vi "SLSC Get Channel Properties.vi"(0 "Node Ptr":T1 format="%.0x", 11 "error in (no error)":errorcluster) -> (2 "Loop time (ms)":u32, 3 "Description":string, 4 "Section Ref out":T1 format="%.0x", 6 "Module Number":i32, 8 "Name":string, 10 "Device Version":string, 13 "Default Value":bool, 14 "Reset Value":bool, 15 "error out":errorcluster)   [LabVIEW 2020, in "SLSC EDS System Explorer.lvlib"]
uses:
  System Explorer/SLSC EDS System Explorer.lvlib
  <vilib>/NI VeriStand/Custom Device API/Custom Device Item Ref.ctl
  Shared/Constants.vi
  <vilib>/NI VeriStand/Custom Device API/Get Item Property (I32).vi
  <vilib>/NI VeriStand/Custom Device API/Get Item Property (Boolean).vi
  <vilib>/NI VeriStand/Custom Device API/Custom Device API.lvlib
  Shared/SLSC EDS Shared.lvlib
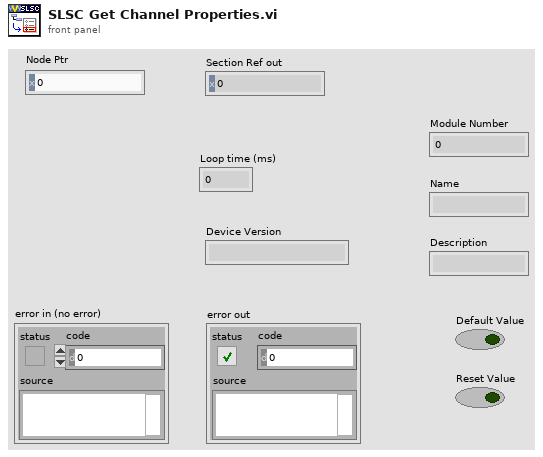
[diagram p1: front panel]
types:
  T1 = typedef "Custom Device API.lvlib/Custom Device Item Ref.ctl" = u64
  T2 = typedef "Custom Device API.lvlib/Custom Device Item Info.ctl" = cluster{"Name":string, "Is Channel":bool, "GUID":string, "Is Waveform":bool}
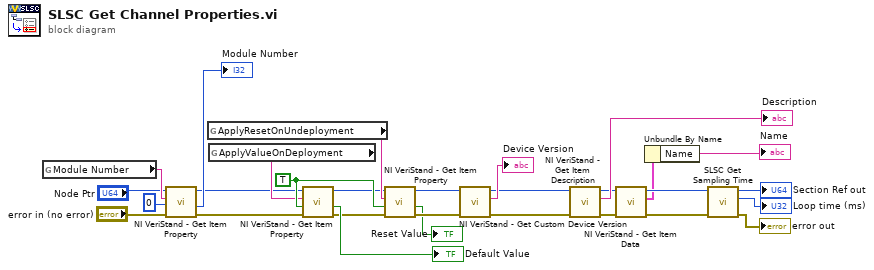
[diagram p0: block diagram]
diagram:
  w22 = TRUE ("Default Value")
  n1 = global read "Constants.vi" "Module Number"() -> (w13:string)
  n2 = call-poly <vilib>:"NI VeriStand - Get Item Property.vi"("error in (no error)"="error in (no error)", "Default Value"=0, "Property Name"=w13, "Item Ref in"="Node Ptr") -> ("error out"=w25:errorcluster, "Value"=→"Module Number":i32, "Item Ref out"=w15:T1)  [unwired: 4 in, 1 out]
  n3 = global read "Constants.vi" "ApplyResetOnUndeployment"() -> (w18:string)
  n4 = global read "Constants.vi" "ApplyValueOnDeployment"() -> (w16:string)
  n5 = call-poly <vilib>:"NI VeriStand - Get Item Property.vi"("error in (no error)"=w25, "Default Value"=w22, "Property Name"=w16, "Item Ref in"=w15) -> ("error out"=w19:errorcluster, "Value"=→"Default Value":bool, "Item Ref out"=w17:T1)  [unwired: 4 in, 1 out]
  n6 = call-poly <vilib>:"NI VeriStand - Get Item Property.vi"("error in (no error)"=w19, "Default Value"=w22, "Property Name"=w18, "Item Ref in"=w17) -> ("error out"=w29:errorcluster, "Value"=→"Reset Value":bool, "Item Ref out"=w28:T1)  [unwired: 4 in, 1 out]
  n7 = call <vilib>:"NI VeriStand - Get Custom Device Version.vi"("error in (no error)"=w29, "Device Ref in"=w28) -> ("error out"=w27:errorcluster, "Value"=→"Device Version":string, "Device Ref out"=w11:T1)  [unwired: 7 in]
  n8 = call <vilib>:"NI VeriStand - Get Item Description.vi"("error in (no error)"=w27, "Item Ref in"=w11) -> ("error out"=w8:errorcluster, "Description"=→"Description":string, "Item Ref out"=w6:T1)  [unwired: 7 out]
  n9 = call <vilib>:"NI VeriStand - Get Item Data.vi"("error in (no error)"=w8, "Item Ref in"=w6) -> ("error out"=w24:errorcluster, "Item Info"=w9:T2, "Item Ref out"=w23:T1)  [unwired: 7 out]
  n10 = Unbundle By Name(w9) -> ("Name"=→"Name":string)
  n11 = call "SLSC Get Sampling Time.vi"("error in (no error)"=w24, "Item Ref in"=w23) -> ("error out"=→"error out":errorcluster, "Loop time (ms)"=→"Loop time (ms)":u32, "Section Ref out"=→"Section Ref out":T1)  [unwired: 7 in]
